vi "Read Pattern Script.vi"(8 "error in (no error)":errorcluster, 11 "SPI_Frame_Root in":refnum<class "SPI_Frame_Root.lvclass">) -> (0 "error out":errorcluster, 2 "Pattern Script":string, 3 "SPI_Frame_Root out":refnum<class "SPI_Frame_Root.lvclass">)   [LabVIEW 2018, in "SPI_Frame_Root.lvclass"]
uses:
  SPI_Frame_Root.lvclass
  SPI_Frame_Root.lvclass/SPI_Frame_Root.ctl
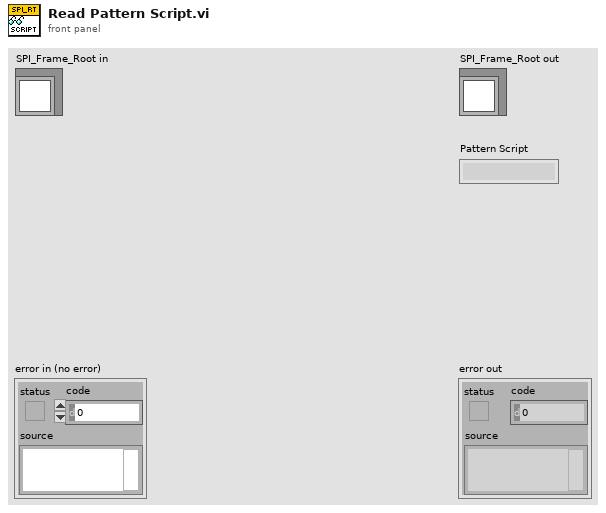
[diagram p1: front panel]
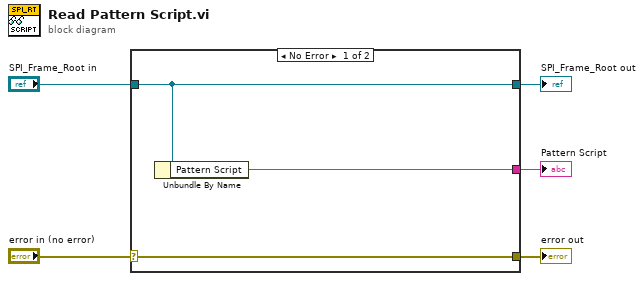
[diagram p0: block diagram]
diagram:
  n1 = case shown="No Error" "error in (no error)" {
    selector: "error in (no error)" -> [w8 w9]
    tunnel: [w8 w9] -> w4
    tunnel: [w7 w10] -> w2
    tunnel: "SPI_Frame_Root in" -> [w7 w10]
    tunnel: [w6 _] -> w1
    frame No Error {
      n2 = Unbundle By Name(w7) -> ("Pattern Script"=w6:string)
    }
    frame Error {
    }
  }
  "error out" <- w4
  "SPI_Frame_Root out" <- w2
  "Pattern Script" <- w1
